vi "stop.vi"(9 "枚举":enum16{"write", "read"}(ring)=enum."read", 11 "停止":bool) -> (3 "停止":bool)   [LabVIEW 2018]
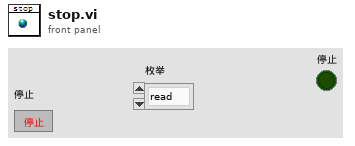
[diagram p1: front panel]
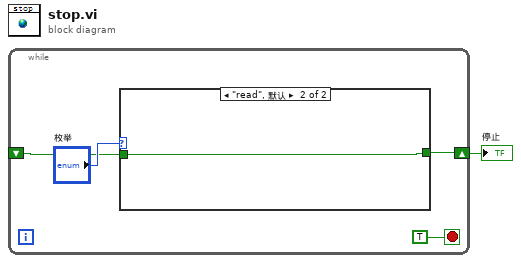
[diagram p0: block diagram]
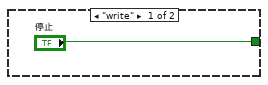
[diagram p2: hidden frame]
diagram:
  n1 = while {
    shift-right: [w3] -> w1
    shift-left: _ -> [w2]
    stop <- TRUE stop-if-true
    n2 = case shown="\"read\", 默认" "枚举" {
      tunnel: ["停止" w7] -> w3
      tunnel: w2 -> [_ w7]
      frame "write" {
      }
      frame "read", Default {
      }
    }
  }
  "停止" <- w1
